vi "FGV Fehlerliste.vi"(6 "Aktionen Fehlerliste":T1) -> (2 "Gespeicherte Fehler":string[](array[string]), 3 "Aktuelle Fehler":string[](array[string]))   [LabVIEW 2020, in "cRIO Ueberwachung.lvlib"]
uses:
  cRIO Ueberwachung.lvlib
  Fehler.ctl
  FGV Fehlerliste Aktionen.ctl
  Allgemein/allgemeine Sub-VIs.lvlib
panel:
  in  "Fehlerliste":T2[](array[typedef]) {"level" items=["Geringfügiger Fehler", "Schwerer Fehler", "Nicht behebbarer Fehler"]}
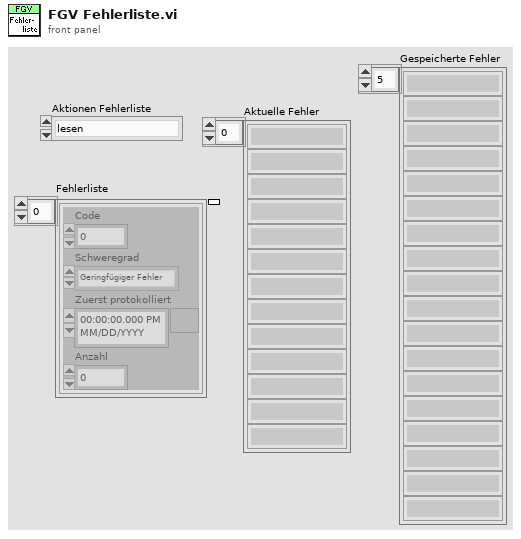
[diagram p1: front panel]
types:
  T1 = typedef "cRIO Ueberwachung.lvlib/FGV Fehlerliste Aktionen.ctl" = enum16{"lesen", "abfragen", "löschen", "laden", "speichern"}
  T2 = typedef "cRIO Ueberwachung.lvlib/Fehler.ctl" = cluster{"code":i32, "level":i32, "first reported time":timestamp, "number reported":u32}
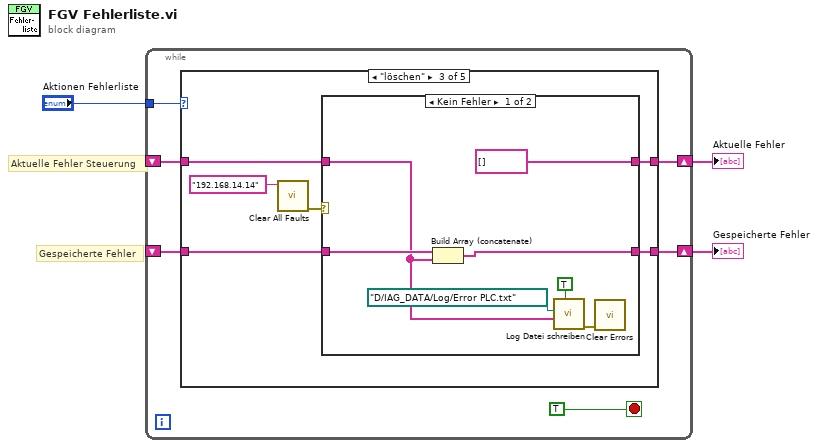
[diagram p0: block diagram]
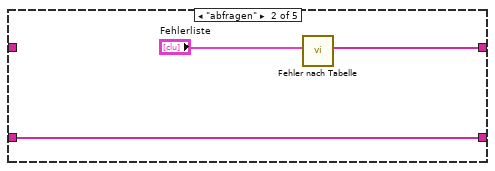
[diagram p3: hidden frame]
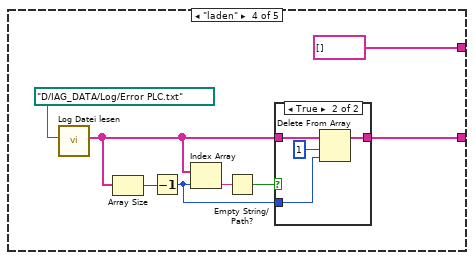
[diagram p5: hidden frame]
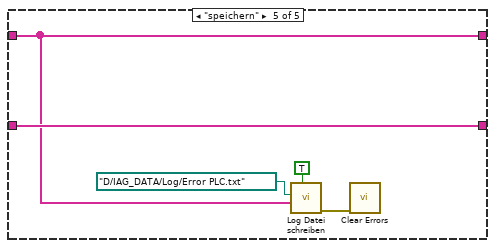
[diagram p7: hidden frame]
diagram:
  # "Gespeicherte Fehler"
  # "Aktuelle Fehler Steuerung"
  n1 = while {
    tunnel: "Aktionen Fehlerliste" -> [w8]
    shift-right: [w7] -> w1
    shift-left: _ -> [w6]
    shift-right: [w5] -> w2
    shift-left: _ -> [w4]
    stop <- TRUE stop-if-true
    n2 = case shown="\"löschen\"" w8 {
      tunnel: [w11 w12 w19 string[] [] ("Tabelle Fehler") w44] -> w7
      tunnel: w6 -> [w11 _ w17 _ w44]
      tunnel: [w10 w14 w15 w31 w45] -> w5
      tunnel: w4 -> [w10 w14 w16 _ w45]
      frame "lesen", Default {
      }
      frame "abfragen" {
        n3 = call "Fehler nach Tabelle.vi"("Fehler"="Fehlerliste") -> ("Tabelle Fehler"=w12:string[])  [unwired: 10 in]
      }
      frame "löschen" {
        n4 = call <vilib>:"Clear All Faults.vi"("target address (localhost)"="192.168.14.14") -> ("error out"=w18:errorcluster)  [unwired: 10 in]
        n5 = case shown="Kein Fehler" w18 {
          tunnel: [string[] [] ("Tabelle Fehler") w29] -> w19
          tunnel: w17 -> [w22 w29]
          tunnel: w16 -> [w26 w28]
          tunnel: [w27 w28] -> w15
          frame No Error {
            n6 = Build Array (concatenate)(w26, w22) -> (w27:string[])
            n7 = call "Log Datei schreiben.vi"("An Datei Anhängen?"=TRUE, "Array"=w22, "Dateipfad"=path "D:/IAG_DATA/Log/Error PLC.txt" ("Datei")) -> ("error out"=w21:errorcluster)  [unwired: 8 in]
            n8 = call <vilib>:"Clear Errors.vi"("error in (no error)"=w21) -> ()  [unwired: 5 in, 2 out]
          }
          frame Error {
          }
        }
      }
      frame "laden" {
        n9 = call "Log Datei lesen.vi"("Dateipfad"=path "D:/IAG_DATA/Log/Error PLC.txt" ("Datei")) -> ("Array"=w32:string[])  [unwired: 10 in]
        n10 = Array Size(array=w32) -> (size(s)=w35:i32)
        n11 = Decrement(x=w35) -> (x-1=w30:i32)
        n12 = Index Array(array=w32, index=w30) -> (element=w34:string)
        n13 = Empty String/Path?(string/path=w34) -> (empty?=w33:bool)
        n14 = case shown="True" w33 {
          tunnel: w32 -> [w38 w42]
          tunnel: [w38 w41] -> w31
          tunnel: w30 -> [_ w40]
          frame False {
          }
          frame True {
            n15 = Delete From Array(array=w42, length=1 ("Länge"), index=w40) -> (array with subset deleted=w41:string[])  [unwired: 1 out]
          }
        }
      }
      frame "speichern" {
        n16 = call "Log Datei schreiben.vi"("An Datei Anhängen?"=TRUE, "Array"=w44, "Dateipfad"=path "D:/IAG_DATA/Log/Error PLC.txt" ("Datei")) -> ("error out"=w43:errorcluster)  [unwired: 8 in]
        n17 = call <vilib>:"Clear Errors.vi"("error in (no error)"=w43) -> ()  [unwired: 5 in, 2 out]
      }
    }
  }
  "Gespeicherte Fehler" <- w2
  "Aktuelle Fehler" <- w1
